vi "main-for-loop.vi"() -> ()   [LabVIEW 2024]
uses:
  controls/digital-output-cluster.ctl
  controls/digitial-input-cluster.ctl
  controls/analog-output-cluster.ctl
  controls/analog-input-cluster.ctl
  controls/thermocouple-input-cluster.ctl
  controls/adam-5000-serial-settings.ctl
  controls/state-enum.ctl
  <vilib>/Instr/_visa.llb/VISA Configure Serial Port (Instr).vi
  <vilib>/Instr/_visa.llb/VISA Flush IO Buffer Mask.ctl
  controls/adam-5000-all-module-datas.ctl
  controls/adam-5000-all-chassis-data.ctl
  controls/adam-5000-module-cmd-ack.ctl
  controls/adam-5000-chassis-cmd-ack.ctl
  controls/adam-module-select-tab.ctl
panel:
  out "response":string
  out "cmd string":string
  out "Ack":bool
  out "Sampling":bool
  in  "Slot 1: Module Type":T1(ring)
  out "slot: 1":T2
  in  "Digital Outputs 2":T3
  out "Digital Inputs 2":T4
  in  "Analog Outputs 2":T5
  out "Analog Inputs 2":T6
  out "Thermocouple Inputs (degC) 2":T7
  out "current-slot":i32
  in  "chassis-slot":i32=5
  out "response":string
  out "cmd string":string
  out "Ack":bool
  out "Sampling":bool
  in  "Slot 0: Module Type":T1(ring)
  out "slot: 0":T2
  in  "Digital Outputs":T3
  out "Digital Inputs":T4
  in  "Analog Outputs":T5
  out "Analog Inputs":T6
  out "Thermocouple Inputs (degC)":T7
  in  "Chassis Settings":T8={"VISA resource name"="COM10", "baud rate (19200)"=19200, "Chassis ID"=1}
  in  "Debug Mode":bool
  out "Loop Time (mS)":u32
  out "Loop Counter":i32
  out "Write Success":bool
  out "error IO":errorcluster
  out "error":errorcluster
  in  "exit":bool
  # "ADAM 5000 Controller"
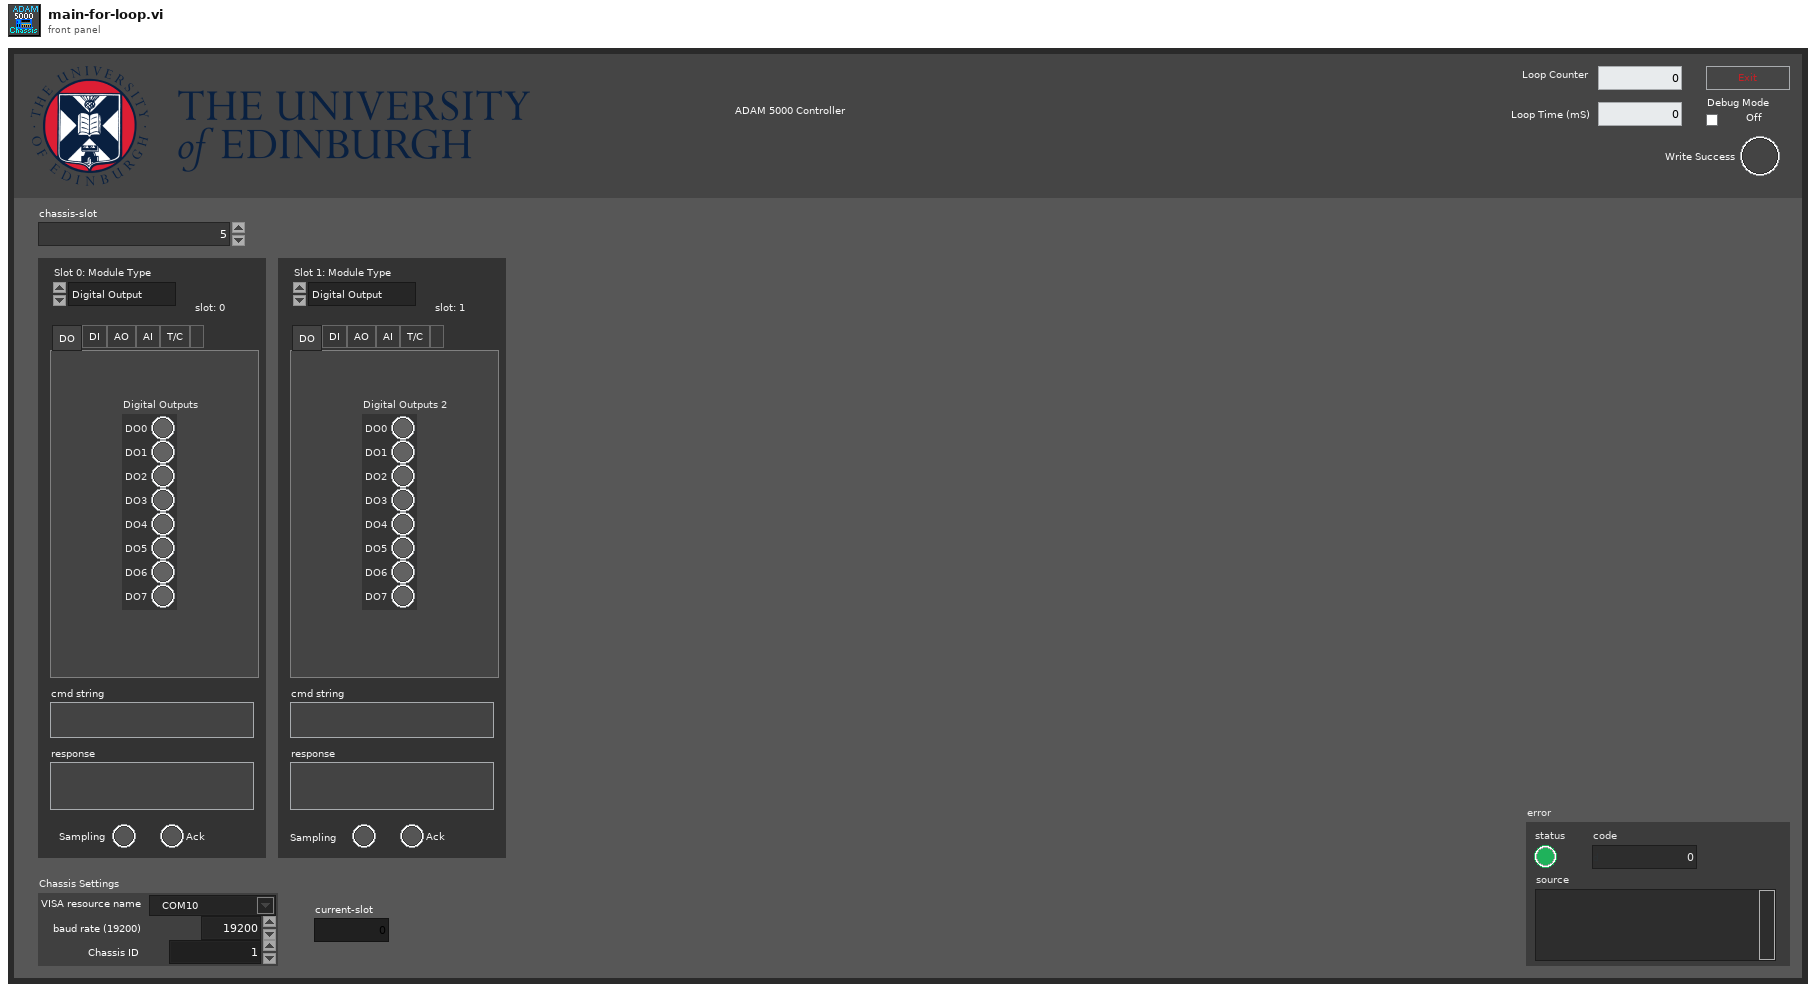
[diagram p1: front panel]
types:
  T1 = enum16{"Digital Output", "Digital Input", "Analog Output", "Analog Input", "Thermocouple", "Power Relay", "empty"}
  T2 = typedef "adam-module-select-tab.ctl" = enum32{"DO", "DI", "AO", "AI", "T/C", ""}
  T3 = typedef "digital-output-cluster.ctl" = cluster{"DO0":bool, "DO1":bool, "DO2":bool, "DO3":bool, "DO4":bool, "DO5":bool, "DO6":bool, "DO7":bool}
  T4 = typedef "digitial-input-cluster.ctl" = cluster{"DI0":bool, "DI1":bool, "DI2":bool, "DI3":bool, "DI4":bool, "DI5":bool, "DI6":bool, "DI7":bool}
  T5 = typedef "analog-output-cluster.ctl" = cluster{"AO0":dbl, "AO1":dbl, "AO2":dbl, "AO3":dbl}
  T6 = typedef "analog-input-cluster.ctl" = cluster{"AO0":dbl, "AO1":dbl, "AO2":dbl, "AO3":dbl, "AO4":dbl, "AO5":dbl, "AO6":dbl, "AO7":dbl}
  T7 = typedef "thermocouple-input-cluster.ctl" = cluster{"TC0":dbl, "TC1":dbl, "TC2":dbl, "TC3":dbl, "TC4":dbl, "TC5":dbl, "TC6":dbl}
  T8 = typedef "adam-5000-serial-settings.ctl" = cluster{"VISA resource name":refnum<visa-resource-name>, "baud rate (19200)":u32, "Chassis ID":u8}
  T9 = typedef "adam-5000-chassis-cmd-ack.ctl" = cluster{"0 cmd-ack":T10, "1 cmd-ack":T10, "2 cmd-ack":T10, "3 cmd-ack":T10, "4 cmd-ack":T10, "5 cmd-ack":T10, "6 cmd-ack":T10, "7 cmd-ack":T10}
  T10 = typedef "adam-5000-module-cmd-ack.ctl" = cluster{"cmd out":string, "acknowledge char":string}
  T11 = typedef "adam-5000-all-chassis-data.ctl" = cluster{"slot:0":T12, "slot:1":T12, "slot:2":T12, "slot:3":T12, "slot:4":T12, "slot:5":T12, "slot:6":T12, "slot:7":T12}
  T12 = typedef "adam-5000-all-module-datas.ctl" = cluster{"Digital Outputs":T3, "Digital Inputs":T4, "Analog Outputs":T5, "Analog Inputs":T6, "Thermocouple Inputs (degC)":T7}
  T13 = typedef "state-enum.ctl" = enum16{"init", "manual", "start", "run", "hold", "stop", ""}
  T14 = cluster{"Slot 0: Module Type":enum16{"Digital Output", "Digital Input", "Analog Output", "Analog Input", "Thermocouple", "Power Relay", "empty"}, "Slot 1: Module Type":enum16{"Digital Output", "Digital Input", "Analog Output", "Analog Input", "Thermocouple", "Power Relay", "empty"}}
  T15 = cluster{"Digital Outputs":T3, "Digital Outputs 2":T3}
  T16 = cluster{"Analog Outputs":T5, "Analog Outputs 2":T5}
  T17 = enum16{"Digital Output", "Digital Input", "Analog Output", "Analog Input", "Thermocouple", "Power Relay", "empty"}[]
  T18 = cluster{"[0]":cluster{"Sampling":bool, "Ack":bool}, "[1]":cluster{"Sampling":bool, "Ack":bool}, "[2]":cluster{"Sampling":bool, "Ack":bool}, "[3]":cluster{"Sampling":bool, "Ack":bool}, "[4]":cluster{"Sampling":bool, "Ack":bool}, "[5]":cluster{"Sampling":bool, "Ack":bool}, "[6]":cluster{"Sampling":bool, "Ack":bool}, "[7]":cluster{"Sampling":bool, "Ack":bool}, "[8]":cluster{"Sampling":bool, "Ack":bool}}
  T19 = cluster{"[0]":T2, "[1]":T2, "[2]":T2, "[3]":T2, "[4]":T2, "[5]":T2, "[6]":T2, "[7]":T2, "[8]":T2}
  T20 = cluster{"[0]":T12, "[1]":T12, "[2]":T12, "[3]":T12, "[4]":T12, "[5]":T12, "[6]":T12, "[7]":T12, "[8]":T12}
  T21 = cluster{"[0]":T10, "[1]":T10, "[2]":T10, "[3]":T10, "[4]":T10, "[5]":T10, "[6]":T10, "[7]":T10, "[8]":T10}
  T22 = typedef "VISA Flush IO Buffer Mask.ctl" = u16
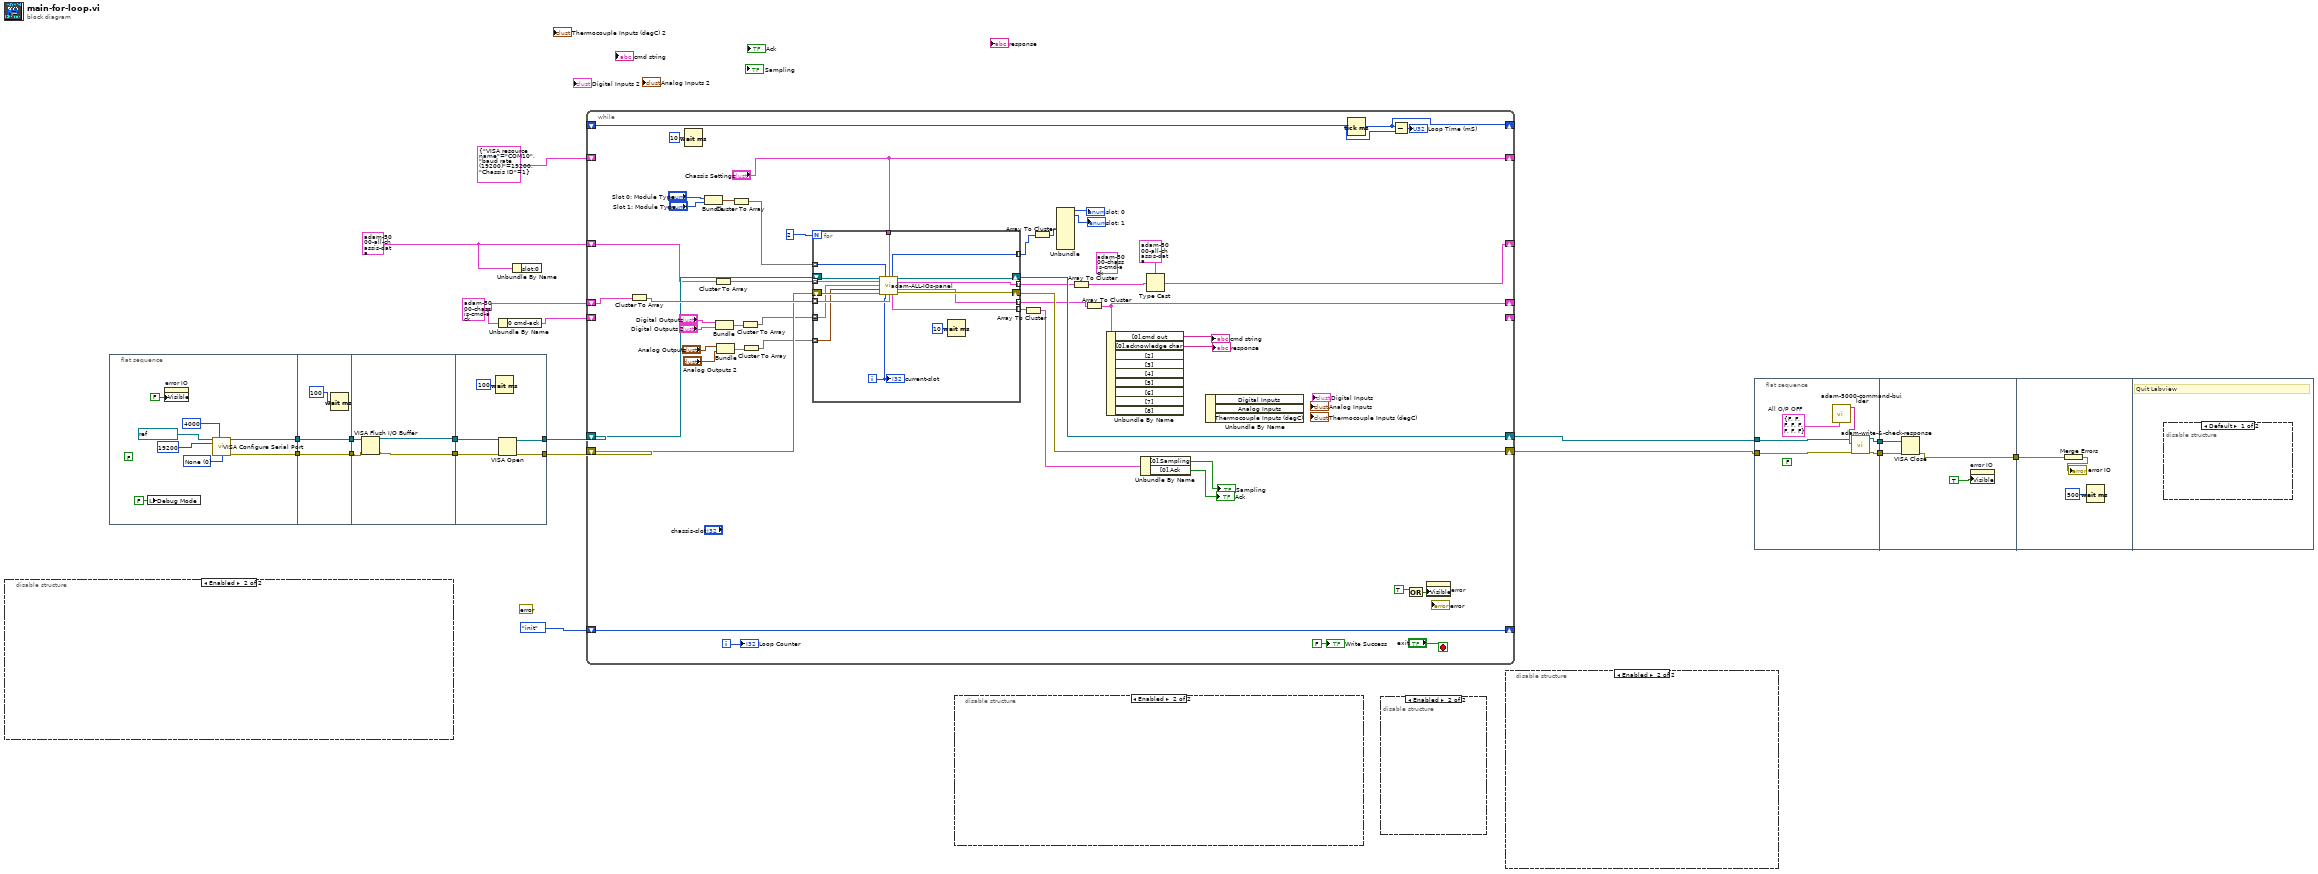
[diagram p0: block diagram]
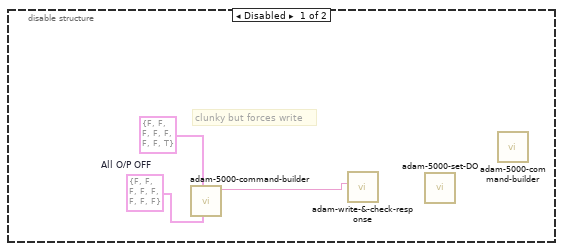
[diagram p2: hidden frame]
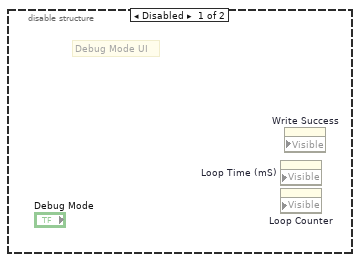
[diagram p3: hidden frame]
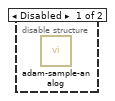
[diagram p4: hidden frame]
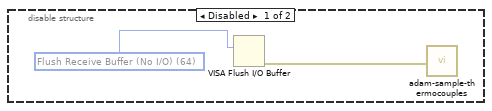
[diagram p5: hidden frame]
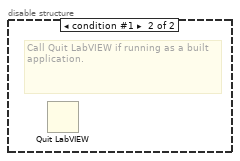
[diagram p6: hidden frame]
diagram:
  w1 = T9 {"0 cmd-ack"={"cmd out"="", "acknowledge char"=""}, "1 cmd-ack"={"cmd out"="", "acknowledge char"=""}, "2 cmd-ack"={"cmd out"="", "acknowledge char"=""}, "3 cmd-ack"={"cmd out"="", "acknowledge char"=""}, "4 cmd-ack"={"cmd out"="", "acknowledge char"=""}, "5 cmd-ack"={"cmd out"="", "acknowledge char"=""}, "6 cmd-ack"={"cmd out"="", "acknowledge char"=""}, "7 cmd-ack"={"cmd out"="", "acknowledge char"=""}} ("adam-chassis-cmd-ack")
  w3 = T11 {"slot:0"={"Digital Outputs"={"DO0"=FALSE, "DO1"=FALSE, "DO2"=FALSE, "DO3"=FALSE, "DO4"=FALSE, "DO5"=FALSE, "DO6"=FALSE, "DO7"=FALSE}, "Digital Inputs"={"DI0"=FALSE, "DI1"=FALSE, "DI2"=FALSE, "DI3"=FALSE, "DI4"=FALSE, "DI5"=FALSE, "DI6"=FALSE, "DI7"=FALSE}, "Analog Outputs"={"AO0"=0.0, "AO1"=0.0, "AO2"=0.0, "AO3"=0.0}, "Analog Inputs"={"AO0"=0.0, "AO1"=0.0, "AO2"=0.0, "AO3"=0.0, "AO4"=0.0, "AO5"=0.0, "AO6"=0.0, "AO7"=0.0}, "Thermocouple Inputs (degC)"={"TC0"=0.0, "TC1"=0.0, "TC2"=0.0, "TC3"=0.0, "TC4"=0.0, "TC5"=0.0, "TC6"=0.0}}, "slot:1"={"Digital Outputs"={"DO0"=FALSE, "DO1"=FALSE, "DO2"=FALSE, "DO3"=FALSE, "DO4"=FALSE, "DO5"=FALSE, "DO6"=FALSE, "DO7"=FALSE}, "Digital Inputs"={"DI0"=FALSE, "DI1"=FALSE, "DI2"=FALSE, "DI3"=FALSE, "DI4"=FALSE, "DI5"=FALSE, "DI6"=FALSE, "DI7"=FALSE}, "Analog Outputs"={"AO0"=0.0, "AO1"=0.0, "AO2"=0.0, "AO3"=0.0}, "Analog Inputs"={"AO0"=0.0, "AO1"=0.0, "AO2"=0.0, "AO3"=0.0, "AO4"=0.0, "AO5"=0.0, "AO6"=0.0, "AO7"=0.0}, "Thermocouple Inputs (degC)"={"TC0"=0.0, "TC1"=0.0, "TC2"=0.0, "TC3"=0.0, "TC4"=0.0, "TC5"=0.0, "TC6"=0.0}}, "slot:2"={"Digital Outputs"={"DO0"=FALSE, "DO1"=FALSE, "DO2"=FALSE, "DO3"=FALSE, "DO4"=FALSE, "DO5"=FALSE, "DO6"=FALSE, "DO7"=FALSE}, "Digital Inputs"={"DI0"=FALSE, "DI1"=FALSE, "DI2"=FALSE, "DI3"=FALSE, "DI4"=FALSE, "DI5"=FALSE, "DI6"=FALSE, "DI7"=FALSE}, "Analog Outputs"={"AO0"=0.0, "AO1"=0.0, "AO2"=0.0, "AO3"=0.0}, "Analog Inputs"={"AO0"=0.0, "AO1"=0.0, "AO2"=0.0, "AO3"=0.0, "AO4"=0.0, "AO5"=0.0, "AO6"=0.0, "AO7"=0.0}, "Thermocouple Inputs (degC)"={"TC0"=0.0, "TC1"=0.0, "TC2"=0.0, "TC3"=0.0, "TC4"=0.0, "TC5"=0.0, "TC6"=0.0}}, "slot:3"={"Digital Outputs"={"DO0"=FALSE, "DO1"=FALSE, "DO2"=FALSE, "DO3"=FALSE, "DO4"=FALSE, "DO5"=FALSE, "DO6"=FALSE, "DO7"=FALSE}, "Digital Inputs"={"DI0"=FALSE, "DI1"=FALSE, "DI2"=FALSE, "DI3"=FALSE, "DI4"=FALSE, "DI5"=FALSE, "DI6"=FALSE, "DI7"=FALSE}, "Analog Outputs"={"AO0"=0.0, "AO1"=0.0, "AO2"=0.0, "AO3"=0.0}, "Analog Inputs"={"AO0"=0.0, "AO1"=0.0, "AO2"=0.0, "AO3"=0.0, "AO4"=0.0, "AO5"=0.0, "AO6"=0.0, "AO7"=0.0}, "Thermocouple Inputs (degC)"={"TC0"=0.0, "TC1"=0.0, "TC2"=0.0, "TC3"=0.0, "TC4"=0.0, "TC5"=0.0, "TC6"=0.0}}, "slot:4"={"Digital Outputs"={"DO0"=FALSE, "DO1"=FALSE, "DO2"=FALSE, "DO3"=FALSE, "DO4"=FALSE, "DO5"=FALSE, "DO6"=FALSE, "DO7"=FALSE}, "Digital Inputs"={"DI0"=FALSE, "DI1"=FALSE, "DI2"=FALSE, "DI3"=FALSE, "DI4"=FALSE, "DI5"=FALSE, "DI6"=FALSE, "DI7"=FALSE}, "Analog Outputs"={"AO0"=0.0, "AO1"=0.0, "AO2"=0.0, "AO3"=0.0}, "Analog Inputs"={"AO0"=0.0, "AO1"=0.0, "AO2"=0.0, "AO3"=0.0, "AO4"=0.0, "AO5"=0.0, "AO6"=0.0, "AO7"=0.0}, "Thermocouple Inputs (degC)"={"TC0"=0.0, "TC1"=0.0, "TC2"=0.0, "TC3"=0.0, "TC4"=0.0, "TC5"=0.0, "TC6"=0.0}}, "slot:5"={"Digital Outputs"={"DO0"=FALSE, "DO1"=FALSE, "DO2"=FALSE, "DO3"=FALSE, "DO4"=FALSE, "DO5"=FALSE, "DO6"=FALSE, "DO7"=FALSE}, "Digital Inputs"={"DI0"=FALSE, "DI1"=FALSE, "DI2"=FALSE, "DI3"=FALSE, "DI4"=FALSE, "DI5"=FALSE, "DI6"=FALSE, "DI7"=FALSE}, "Analog Outputs"={"AO0"=0.0, "AO1"=0.0, "AO2"=0.0, "AO3"=0.0}, "Analog Inputs"={"AO0"=0.0, "AO1"=0.0, "AO2"=0.0, "AO3"=0.0, "AO4"=0.0, "AO5"=0.0, "AO6"=0.0, "AO7"=0.0}, "Thermocouple Inputs (degC)"={"TC0"=0.0, "TC1"=0.0, "TC2"=0.0, "TC3"=0.0, "TC4"=0.0, "TC5"=0.0, "TC6"=0.0}}, "slot:6"={"Digital Outputs"={"DO0"=FALSE, "DO1"=FALSE, "DO2"=FALSE, "DO3"=FALSE, "DO4"=FALSE, "DO5"=FALSE, "DO6"=FALSE, "DO7"=FALSE}, "Digital Inputs"={"DI0"=FALSE, "DI1"=FALSE, "DI2"=FALSE, "DI3"=FALSE, "DI4"=FALSE, "DI5"=FALSE, "DI6"=FALSE, "DI7"=FALSE}, "Analog Outputs"={"AO0"=0.0, "AO1"=0.0, "AO2"=0.0, "AO3"=0.0}, "Analog Inputs"={"AO0"=0.0, "AO1"=0.0, "AO2"=0.0, "AO3"=0.0, "AO4"=0.0, "AO5"=0.0, "AO6"=0.0, "AO7"=0.0}, "Thermocouple Inputs (degC)"={"TC0"=0.0, "TC1"=0.0, "TC2"=0.0, "TC3"=0.0, "TC4"=0.0, "TC5"=0.0, "TC6"=0.0}}, "slot:7"={"Digital Outputs"={"DO0"=FALSE, "DO1"=FALSE, "DO2"=FALSE, "DO3"=FALSE, "DO4"=FALSE, "DO5"=FALSE, "DO6"=FALSE, "DO7"=FALSE}, "Digital Inputs"={"DI0"=FALSE, "DI1"=FALSE, "DI2"=FALSE, "DI3"=FALSE, "DI4"=FALSE, "DI5"=FALSE, "DI6"=FALSE, "DI7"=FALSE}, "Analog Outputs"={"AO0"=0.0, "AO1"=0.0, "AO2"=0.0, "AO3"=0.0}, "Analog Inputs"={"AO0"=0.0, "AO1"=0.0, "AO2"=0.0, "AO3"=0.0, "AO4"=0.0, "AO5"=0.0, "AO6"=0.0, "AO7"=0.0}, "Thermocouple Inputs (degC)"={"TC0"=0.0, "TC1"=0.0, "TC2"=0.0, "TC3"=0.0, "TC4"=0.0, "TC5"=0.0, "TC6"=0.0}}}
  (unwired) errorcluster {"status"=FALSE, "code"=0, "source"=""} ("error")
  n1 = disable-structure shown="Enabled" {
    frame Disabled {
      w21 = T3 {"DO0"=FALSE, "DO1"=FALSE, "DO2"=FALSE, "DO3"=FALSE, "DO4"=FALSE, "DO5"=FALSE, "DO6"=FALSE, "DO7"=FALSE}  # All O/P OFF
      # "clunky but forces write"
      n2 = call "adam-5000-command-builder.vi"("Output Control"=w21, "Current Output State"=T3 {"DO0"=FALSE, "DO1"=FALSE, "DO2"=FALSE, "DO3"=FALSE, "DO4"=FALSE, "DO5"=FALSE, "DO6"=FALSE, "DO7"=TRUE}) -> ("Command Out"=w20:string)  [unwired: 7 in, 2 out]
      n3 = call "adam-write-&-check-response.vi"("write buffer"=w20) -> ("VISA resource name"=w19:refnum<visa-resource-name>)  [unwired: 4 in, 6 out]
      n4 = call "adam-5000-set-DO.vi"() -> ()  [unwired: 6 in, 6 out]
      n5 = call "adam-5000-command-builder.vi"() -> ()  [unwired: 9 in, 3 out]
    }
    frame Enabled {
    }
  }
  n6 = flat-sequence {
    tunnel: [w29] -> w12
    tunnel: [w28] -> w11
    tunnel: w12 -> [w33]
    tunnel: [w33] -> w10
    tunnel: w11 -> [w32]
    tunnel: [w32] -> w9
    tunnel: w10 -> [w37]
    tunnel: [w35] -> w8
    tunnel: w9 -> [w36]
    tunnel: [w34] -> w7
    tunnel: w8 -> [w41]
    tunnel: w7 -> [w40]
    tunnel: [w39] -> w6
    tunnel: [w38] -> w5
    frame #0 {
      w26 = u16 0 items=["None", "XON/XOFF", "RTS/CTS", "XON/XOFF & RTS/CTS", "DTR/DSR", "XON/XOFF & DTR/DSR"] ("flow control (0:none)")
      (unwired) FALSE ("V1")
      n7 = local write "Debug Mode"(FALSE ("Debug Mode")) -> ()
      n8 = property on="error IO" class="Clust (strict)"("Visible"=FALSE) -> ()  [unwired: 2 in, 2 out]
      n9 = call-poly "VISA Configure Serial Port"("VISA resource name"=refnum<visa-resource-name> "COM10", "timeout (10sec)"=u32 4000, "baud rate (9600)"=u32 19200, "flow control (0:none)"=w26) -> ("VISA resource name out"=w29:refnum<visa-resource-name>, "error out"=w28:errorcluster)  [unwired: 10 in]
    }
    frame #1 {
      n10 = Wait (ms)(milliseconds to wait=u32 100) -> ()  [unwired: 1 out]
    }
    frame #2 {
      n11 = VISA Flush I/O Buffer(VISA resource name=w37, error in (no error)=w36) -> (VISA resource name out=w35:refnum<visa-resource-name>, error out=w34:errorcluster)  [unwired: 1 in]
    }
    frame #3 {
      n12 = Wait (ms)(milliseconds to wait=u32 100) -> ()  [unwired: 1 out]
      n13 = VISA Open(error in (no error)=w40, VISA resource name=w41) -> (VISA resource name=w39:refnum<visa-resource-name>, error out=w38:errorcluster)  [unwired: 3 in]
    }
  }
  n14 = Unbundle By Name(w1) -> ("0 cmd-ack"=w2:T10)
  n15 = Unbundle By Name(w3) -> ()  [unwired: 1 out]
  n16 = while {
    shift-right: [w83] -> _
    shift-left: state-enum."init" ("state-enum") -> [w83]
    shift-right: [w57] -> w17
    shift-left: w5 -> [w67]
    shift-right: [w86] -> _
    shift-left: _ -> [w88]
    shift-right: ["Chassis Settings"] -> _
    shift-left: T8 {"VISA resource name"="COM10", "baud rate (19200)"=19200, "Chassis ID"=1} ("Chassis Settings") -> [_]
    shift-right: [w58] -> w4
    shift-left: w6 -> [w73]
    shift-right: _ -> [_]
    shift-left: w2 -> [_]
    shift-right: [w47] -> _
    shift-left: w3 -> [w49]
    shift-right: [w43] -> _
    shift-left: w1 -> [w79]
    i -> [w89]
    stop <- "exit" stop-if-true
    w44 = T9 {"0 cmd-ack"={"cmd out"="", "acknowledge char"=""}, "1 cmd-ack"={"cmd out"="", "acknowledge char"=""}, "2 cmd-ack"={"cmd out"="", "acknowledge char"=""}, "3 cmd-ack"={"cmd out"="", "acknowledge char"=""}, "4 cmd-ack"={"cmd out"="", "acknowledge char"=""}, "5 cmd-ack"={"cmd out"="", "acknowledge char"=""}, "6 cmd-ack"={"cmd out"="", "acknowledge char"=""}, "7 cmd-ack"={"cmd out"="", "acknowledge char"=""}} ("adam-chassis-cmd-ack")
    n17 = Cluster To Array(cluster=w79) -> (array=w78:T10[])
    n18 = Wait (ms)(milliseconds to wait=u32 10) -> ()  [unwired: 1 out]
    n19 = Bundle("Slot 0: Module Type"="Slot 0: Module Type", "Slot 1: Module Type"="Slot 1: Module Type") -> (w75:T14)  [unwired: 1 in]
    n20 = Cluster To Array(cluster=w49) -> (array=w80:T12[])
    n21 = Bundle("Digital Outputs"="Digital Outputs", "Digital Outputs 2"="Digital Outputs 2") -> (w66:T15)  [unwired: 1 in]
    n22 = Bundle("Analog Outputs"="Analog Outputs", "Analog Outputs 2"="Analog Outputs 2") -> (w60:T16)  [unwired: 1 in]
    n23 = Cluster To Array(cluster=w75) -> (array=w74:T17)
    n24 = Cluster To Array(cluster=w66) -> (array=w63:T3[])
    n25 = Cluster To Array(cluster=w60) -> (array=w59:T5[])
    n26 = for {
      N: 2 -> [_]
      tunnel: w80 -> [w106] mode=indexing
      tunnel: w78 -> [w105] mode=indexing
      tunnel: w74 -> [w103] mode=indexing
      tunnel: [w100] -> w70 mode=indexing
      tunnel: "Chassis Settings" -> [w99]
      shift-right: [w97] -> w57
      shift-left: w67 -> [w98]
      shift-right: [w101] -> w58
      shift-left: w73 -> [w102]
      tunnel: [w96] -> _ mode=indexing
      tunnel: w63 -> [w96] mode=indexing
      tunnel: w59 -> [w95] mode=indexing
      tunnel: [w92] -> w56 mode=indexing
      tunnel: [w94] -> w50 mode=indexing
      tunnel: [w93] -> w46 mode=indexing
      i -> [w104]
      n27 = call "adam-ALL-IOs-panel.vi"("VISA Refnum in"=w102, "Module Type"=w103, "Chassis Settings"=w99, "ADAM-5000-data-current"=w106, "Digital Outputs"=w96, "Analog Outputs"=w95, "error in (no error)"=w98, "chassis-slot"=w104, "cmd-ack-in"=w105) -> ("slot: 0"=w100:T2, "VISA Refnum out"=w101:refnum<visa-resource-name>, "ADAM-5000-data-new"=w94:T12, "cmd-ack-out"=w93:T10, "status-cluster"=w92:cluster{"Sampling":bool, "Ack":bool}, "error out"=w97:errorcluster)  [unwired: 1 in]
      n28 = Wait (ms)(milliseconds to wait=u32 10) -> ()  [unwired: 1 out]
      "current-slot" <- w104
    }
    n29 = Array To Cluster(array=w56) -> (cluster=w55:T18)
    n30 = Array To Cluster(array=w70) -> (cluster=w69:T19)
    n31 = Unbundle(w69) -> ("[0]"=→"slot: 0":T2, "[1]"=→"slot: 1":T2)  [unwired: 7 out]
    n32 = Array To Cluster(array=w50) -> (cluster=w48:T20)
    n33 = Array To Cluster(array=w46) -> (cluster=w43:T21)
    n34 = Unbundle By Name(w43) -> ("[0].cmd out"=→"cmd string":string, "[0].acknowledge char"=→"response":string)  [unwired: 7 out]
    n35 = Unbundle By Name(w55) -> ("[0].Sampling"=→"Sampling":bool, "[0].Ack"=→"Ack":bool)
    n36 = Type Cast(type=T11 {"slot:0"={"Digital Outputs"={"DO0"=FALSE, "DO1"=FALSE, "DO2"=FALSE, "DO3"=FALSE, "DO4"=FALSE, "DO5"=FALSE, "DO6"=FALSE, "DO7"=FALSE}, "Digital Inputs"={"DI0"=FALSE, "DI1"=FALSE, "DI2"=FALSE, "DI3"=FALSE, "DI4"=FALSE, "DI5"=FALSE, "DI6"=FALSE, "DI7"=FALSE}, "Analog Outputs"={"AO0"=0.0, "AO1"=0.0, "AO2"=0.0, "AO3"=0.0}, "Analog Inputs"={"AO0"=0.0, "AO1"=0.0, "AO2"=0.0, "AO3"=0.0, "AO4"=0.0, "AO5"=0.0, "AO6"=0.0, "AO7"=0.0}, "Thermocouple Inputs (degC)"={"TC0"=0.0, "TC1"=0.0, "TC2"=0.0, "TC3"=0.0, "TC4"=0.0, "TC5"=0.0, "TC6"=0.0}}, "slot:1"={"Digital Outputs"={"DO0"=FALSE, "DO1"=FALSE, "DO2"=FALSE, "DO3"=FALSE, "DO4"=FALSE, "DO5"=FALSE, "DO6"=FALSE, "DO7"=FALSE}, "Digital Inputs"={"DI0"=FALSE, "DI1"=FALSE, "DI2"=FALSE, "DI3"=FALSE, "DI4"=FALSE, "DI5"=FALSE, "DI6"=FALSE, "DI7"=FALSE}, "Analog Outputs"={"AO0"=0.0, "AO1"=0.0, "AO2"=0.0, "AO3"=0.0}, "Analog Inputs"={"AO0"=0.0, "AO1"=0.0, "AO2"=0.0, "AO3"=0.0, "AO4"=0.0, "AO5"=0.0, "AO6"=0.0, "AO7"=0.0}, "Thermocouple Inputs (degC)"={"TC0"=0.0, "TC1"=0.0, "TC2"=0.0, "TC3"=0.0, "TC4"=0.0, "TC5"=0.0, "TC6"=0.0}}, "slot:2"={"Digital Outputs"={"DO0"=FALSE, "DO1"=FALSE, "DO2"=FALSE, "DO3"=FALSE, "DO4"=FALSE, "DO5"=FALSE, "DO6"=FALSE, "DO7"=FALSE}, "Digital Inputs"={"DI0"=FALSE, "DI1"=FALSE, "DI2"=FALSE, "DI3"=FALSE, "DI4"=FALSE, "DI5"=FALSE, "DI6"=FALSE, "DI7"=FALSE}, "Analog Outputs"={"AO0"=0.0, "AO1"=0.0, "AO2"=0.0, "AO3"=0.0}, "Analog Inputs"={"AO0"=0.0, "AO1"=0.0, "AO2"=0.0, "AO3"=0.0, "AO4"=0.0, "AO5"=0.0, "AO6"=0.0, "AO7"=0.0}, "Thermocouple Inputs (degC)"={"TC0"=0.0, "TC1"=0.0, "TC2"=0.0, "TC3"=0.0, "TC4"=0.0, "TC5"=0.0, "TC6"=0.0}}, "slot:3"={"Digital Outputs"={"DO0"=FALSE, "DO1"=FALSE, "DO2"=FALSE, "DO3"=FALSE, "DO4"=FALSE, "DO5"=FALSE, "DO6"=FALSE, "DO7"=FALSE}, "Digital Inputs"={"DI0"=FALSE, "DI1"=FALSE, "DI2"=FALSE, "DI3"=FALSE, "DI4"=FALSE, "DI5"=FALSE, "DI6"=FALSE, "DI7"=FALSE}, "Analog Outputs"={"AO0"=0.0, "AO1"=0.0, "AO2"=0.0, "AO3"=0.0}, "Analog Inputs"={"AO0"=0.0, "AO1"=0.0, "AO2"=0.0, "AO3"=0.0, "AO4"=0.0, "AO5"=0.0, "AO6"=0.0, "AO7"=0.0}, "Thermocouple Inputs (degC)"={"TC0"=0.0, "TC1"=0.0, "TC2"=0.0, "TC3"=0.0, "TC4"=0.0, "TC5"=0.0, "TC6"=0.0}}, "slot:4"={"Digital Outputs"={"DO0"=FALSE, "DO1"=FALSE, "DO2"=FALSE, "DO3"=FALSE, "DO4"=FALSE, "DO5"=FALSE, "DO6"=FALSE, "DO7"=FALSE}, "Digital Inputs"={"DI0"=FALSE, "DI1"=FALSE, "DI2"=FALSE, "DI3"=FALSE, "DI4"=FALSE, "DI5"=FALSE, "DI6"=FALSE, "DI7"=FALSE}, "Analog Outputs"={"AO0"=0.0, "AO1"=0.0, "AO2"=0.0, "AO3"=0.0}, "Analog Inputs"={"AO0"=0.0, "AO1"=0.0, "AO2"=0.0, "AO3"=0.0, "AO4"=0.0, "AO5"=0.0, "AO6"=0.0, "AO7"=0.0}, "Thermocouple Inputs (degC)"={"TC0"=0.0, "TC1"=0.0, "TC2"=0.0, "TC3"=0.0, "TC4"=0.0, "TC5"=0.0, "TC6"=0.0}}, "slot:5"={"Digital Outputs"={"DO0"=FALSE, "DO1"=FALSE, "DO2"=FALSE, "DO3"=FALSE, "DO4"=FALSE, "DO5"=FALSE, "DO6"=FALSE, "DO7"=FALSE}, "Digital Inputs"={"DI0"=FALSE, "DI1"=FALSE, "DI2"=FALSE, "DI3"=FALSE, "DI4"=FALSE, "DI5"=FALSE, "DI6"=FALSE, "DI7"=FALSE}, "Analog Outputs"={"AO0"=0.0, "AO1"=0.0, "AO2"=0.0, "AO3"=0.0}, "Analog Inputs"={"AO0"=0.0, "AO1"=0.0, "AO2"=0.0, "AO3"=0.0, "AO4"=0.0, "AO5"=0.0, "AO6"=0.0, "AO7"=0.0}, "Thermocouple Inputs (degC)"={"TC0"=0.0, "TC1"=0.0, "TC2"=0.0, "TC3"=0.0, "TC4"=0.0, "TC5"=0.0, "TC6"=0.0}}, "slot:6"={"Digital Outputs"={"DO0"=FALSE, "DO1"=FALSE, "DO2"=FALSE, "DO3"=FALSE, "DO4"=FALSE, "DO5"=FALSE, "DO6"=FALSE, "DO7"=FALSE}, "Digital Inputs"={"DI0"=FALSE, "DI1"=FALSE, "DI2"=FALSE, "DI3"=FALSE, "DI4"=FALSE, "DI5"=FALSE, "DI6"=FALSE, "DI7"=FALSE}, "Analog Outputs"={"AO0"=0.0, "AO1"=0.0, "AO2"=0.0, "AO3"=0.0}, "Analog Inputs"={"AO0"=0.0, "AO1"=0.0, "AO2"=0.0, "AO3"=0.0, "AO4"=0.0, "AO5"=0.0, "AO6"=0.0, "AO7"=0.0}, "Thermocouple Inputs (degC)"={"TC0"=0.0, "TC1"=0.0, "TC2"=0.0, "TC3"=0.0, "TC4"=0.0, "TC5"=0.0, "TC6"=0.0}}, "slot:7"={"Digital Outputs"={"DO0"=FALSE, "DO1"=FALSE, "DO2"=FALSE, "DO3"=FALSE, "DO4"=FALSE, "DO5"=FALSE, "DO6"=FALSE, "DO7"=FALSE}, "Digital Inputs"={"DI0"=FALSE, "DI1"=FALSE, "DI2"=FALSE, "DI3"=FALSE, "DI4"=FALSE, "DI5"=FALSE, "DI6"=FALSE, "DI7"=FALSE}, "Analog Outputs"={"AO0"=0.0, "AO1"=0.0, "AO2"=0.0, "AO3"=0.0}, "Analog Inputs"={"AO0"=0.0, "AO1"=0.0, "AO2"=0.0, "AO3"=0.0, "AO4"=0.0, "AO5"=0.0, "AO6"=0.0, "AO7"=0.0}, "Thermocouple Inputs (degC)"={"TC0"=0.0, "TC1"=0.0, "TC2"=0.0, "TC3"=0.0, "TC4"=0.0, "TC5"=0.0, "TC6"=0.0}}}, x=w48) -> (*(type *) &x=w47:T11)
    n37 = Unbundle By Name() -> ()  [unwired: 1 in, 3 out]
    n38 = Tick Count (ms)() -> (millisecond timer value=w86:u32)
    n39 = Subtract(x=w86, y=w88) -> (x-y=→"Loop Time (mS)":u32)
    n40 = Or(x=TRUE ("Debug Mode")) -> (x .or. y?=w85:bool)  [unwired: 1 in]
    n41 = property on="error" class="Clust (strict)"("Visible"=w85) -> ()  [unwired: 2 in, 2 out]
    "Write Success" <- FALSE ("Write Success")
    "Loop Counter" <- w89
  }
  n42 = disable-structure shown="Enabled" {
    frame Disabled {
      w112 = T22 64 items=["Flush Receive Buffer"=16, "Write Transmit Buffer to Device"=32, "Flush Receive Buffer (No I/O)"=64, "Flush Transmit Buffer"=128] ("Mask")
      n43 = VISA Flush I/O Buffer(mask (16)=w112) -> (error out=w111:errorcluster)  [unwired: 2 in, 1 out]
      n44 = call "adam-sample-thermocouples.vi"("error in (no error)"=w111) -> ("status"=w109:string, "read buffer"=w108:string, "acknowledge char"=w110:string)  [unwired: 5 in, 3 out]
    }
    frame Enabled {
    }
  }
  n45 = disable-structure shown="Enabled" {
    frame Disabled {
      n46 = call "adam-sample-analog.vi"() -> ()  [unwired: 6 in, 6 out]
    }
    frame Enabled {
    }
  }
  n47 = disable-structure shown="Enabled" {
    frame Disabled {
      # "Debug Mode UI"
      n48 = property on="Loop Time (mS)" class="DigNum (strict)" props=["Visible"]() -> ()  [unwired: 3 in, 2 out]
      n49 = property on="Loop Counter" class="DigNum (strict)" props=["Visible"]() -> ()  [unwired: 3 in, 2 out]
      n50 = property on="Write Success" class="Bool (strict)" props=["Visible"]() -> ()  [unwired: 3 in, 2 out]
    }
    frame Enabled {
    }
  }
  n51 = flat-sequence {
    tunnel: w17 -> [w118]
    tunnel: [w117] -> w15
    tunnel: [w116] -> w14
    tunnel: w4 -> [w114]
    tunnel: [w120] -> w16
    tunnel: w15 -> [w121]
    tunnel: w14 -> [w122]
    tunnel: w16 -> [w124]
    frame #0 {
      (unwired) FALSE ("V1")
      w115 = T3 {"DO0"=FALSE, "DO1"=FALSE, "DO2"=FALSE, "DO3"=FALSE, "DO4"=FALSE, "DO5"=FALSE, "DO6"=FALSE, "DO7"=FALSE}  # All O/P OFF
      n52 = call "adam-5000-command-builder.vi"("Output Control"=w115) -> ("Command Out"=w119:string)  [unwired: 8 in, 2 out]
      n53 = call "adam-write-&-check-response.vi"("error in (no error)"=w118, "write buffer"=w119, "VISA resource name"=w114) -> ("error out"=w116:errorcluster, "VISA resource name out"=w117:refnum<visa-resource-name>)  [unwired: 3 in, 4 out]
    }
    frame #1 {
      n54 = VISA Close(VISA resource name=w121, error in (no error)=w122) -> (error out=w120:errorcluster)
      n55 = property on="error IO" class="Clust (strict)"("Visible"=TRUE) -> ()  [unwired: 2 in, 2 out]
    }
    frame #2 {
      n56 = Merge Errors(w124) -> (→"error IO":errorcluster)
      n57 = Wait (ms)(milliseconds to wait=u32 500) -> ()  [unwired: 1 out]
    }
    frame #3 {
      # "Quit Labview"
      n58 = disable-structure "Conditional Disable Structure" shown="Default" {
        frame condition #0 (active) {
        }
        frame condition #1 {
          # "Call Quit LabVIEW if running as a built application."
          n59 = Quit LabVIEW() -> ()  [unwired: 1 in]
        }
      }
    }
  }
